vi "1B_AnalyzeAmplitudeRamp_LimitsGraph_sub.vi"(0 "Trimmed Elapsed time from Active Stim ( sec )":dbl[](array[numeric]), 2 "Target":dbl[](array[numeric]), 3 "Tol [ A ]":dbl, 4 "Meas.":dbl[](array[numeric])) -> (7 "Array":T1(array[cluster]), 9 "mean error":dbl format="%#.0p")   [LabVIEW 2010]
uses:
  <vilib>/Analysis/NI_AALBase.lvlib
panel:
  out "variance":dbl format="%#.0p"
  out "std. dev.":dbl format="%#.0p"
  out "Error ( i.e. Meas - Target )":dbl[](array[numeric]) format="%#.0p"
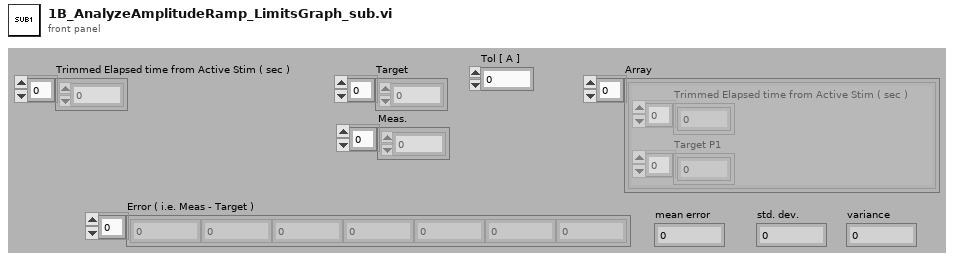
[diagram p1: front panel]
types:
  T1 = cluster{"Trimmed Elapsed time from Active Stim ( sec )":dbl[], "Target P1":dbl[]}[]
  T2 = cluster{"Trimmed Elapsed time from Active Stim ( sec )":dbl[], dbl[]}
  T3 = cluster{"Trimmed Elapsed time from Active Stim ( sec )":dbl[], "Meas.":dbl[]}
  T4 = cluster{"Trimmed Elapsed time from Active Stim ( sec )":dbl[], "Target":dbl[]}
  T5 = cluster{"Trimmed Elapsed time from Active Stim ( sec )":dbl[], "Meas.":dbl[]}[]
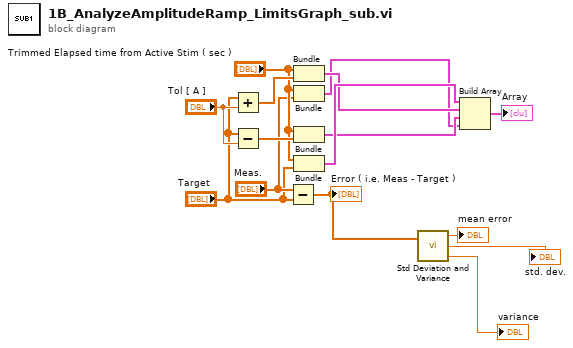
[diagram p0: block diagram]
diagram:
  n1 = Add(x="Target", y="Tol [ A ]") -> (x+y=w13:dbl[])
  n2 = Subtract(x="Target", y="Tol [ A ]") -> (x-y=w14:dbl[])
  n3 = Subtract(x="Meas.", y="Target") -> (x-y=w4:dbl[])
  "Error ( i.e. Meas - Target )" <- w4
  n4 = Bundle("Trimmed Elapsed time from Active Stim ( sec )"="Trimmed Elapsed time from Active Stim ( sec )", w13) -> (w9:T2)  [unwired: 1 in]
  n5 = Bundle("Trimmed Elapsed time from Active Stim ( sec )"="Trimmed Elapsed time from Active Stim ( sec )", "Meas."="Meas.") -> (w7:T3)  [unwired: 1 in]
  n6 = Bundle("Trimmed Elapsed time from Active Stim ( sec )"="Trimmed Elapsed time from Active Stim ( sec )", w14) -> (w8:T2)  [unwired: 1 in]
  n7 = Bundle("Trimmed Elapsed time from Active Stim ( sec )"="Trimmed Elapsed time from Active Stim ( sec )", "Target"="Target") -> (w10:T4)  [unwired: 1 in]
  n8 = call <vilib>:"Std Deviation and Variance.vi"("X"=w4) -> ("mean"=→"mean error":dbl, "standard deviation"=→"std. dev.":dbl, "variance"=→"variance":dbl)  [unwired: 1 in]
  n9 = Build Array(w10, w9, w8, w7) -> (→"Array":T5)
